vi "File - size rollover.vi"(8 "error in (no error)":errorcluster) -> (0 "error out":errorcluster)   [LabVIEW 2026, in "Tests.lvlib"]
doc: "Integration test (Caraya). Verifies a statement logged through the Logger reaches a single registered appender. Launches a manager with the default file disabled and a queue-mode relay capture probe (Open Test Mgr), logs one INFO statement, dequeues from the capture queue with a timeout, and asserts it was delivered and its message matches. Tears down with Close Test Mgr regardless of assertion outcome (SRS-LMBR-019). Uses the manager fixture; no temp root needed.\n\nImplements LMBR-T-039 -> SRS-033. Assert-level IDs: Test-ID-Assert-Checklist.md."
uses:
  Tests.lvlib
  src/TypeDefs/Severity.ctl
  src/TypeDefs/FileAppenderConfig.ctl
  src/TypeDefs/AppenderConfig.ctl
  src/TypeDefs/Filter.ctl
  src/TypeDefs/FilterMode.ctl
  src/TypeDefs/DropPolicy.ctl
  src/TypeDefs/FileConfig.ctl
  <vilib>/addons/_JKI Toolkits/Caraya/classes/Assert/Assert Less_Variant.vi
  <vilib>/addons/_JKI Toolkits/Caraya/classes/Assert/Assert Equal Value_Variant.vi
  <vilib>/addons/_JKI Toolkits/Caraya/classes/Assert/Assert True.vi
  <vilib>/addons/_JKI Toolkits/Caraya/classes/Test/Test.lvclass
  src/Lumberjack.lvlib
  src/Public/Logger.lvclass/Logger.lvclass
  <vilib>/addons/_JKI Toolkits/Caraya/classes/Assert/Assert.lvclass
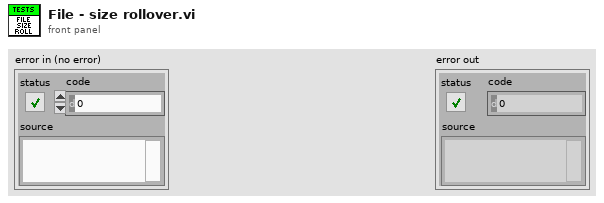
[diagram p1: front panel]
types:
  T1 = typedef "Lumberjack.lvlib/Severity.ctl" = enum16{"OFF", "FATAL", "ERROR", "WARN", "INFO", "DEBUG", "TRACE", "ALL"}
  T2 = typedef "Lumberjack.lvlib/FileAppenderConfig.ctl" = cluster{"common":T3, "file":T7}
  T3 = typedef "Lumberjack.lvlib/AppenderConfig.ctl" = cluster{"id":string, "threshold":T1, "filter":T4, "queueBound":i32, "dropPolicy":T6, "useUTC":bool}
  T4 = typedef "Lumberjack.lvlib/Filter.ctl" = cluster{"mode":T5, "levelMin":T1, "levelMax":T1, "tagPrefix":string}
  T5 = typedef "Lumberjack.lvlib/FilterMode.ctl" = enum16{"Mirror", "Routed"}
  T6 = typedef "Lumberjack.lvlib/DropPolicy.ctl" = enum16{"DropOldest", "DropNewest", "LevelAware"}
  T7 = typedef "Lumberjack.lvlib/FileConfig.ctl" = cluster{"rootFolder":path, "maxFileSize":i64, "maxFileCount":i32, "baseName":string, "extension":string, "delimiter":string, "calendarFolderTree":bool}
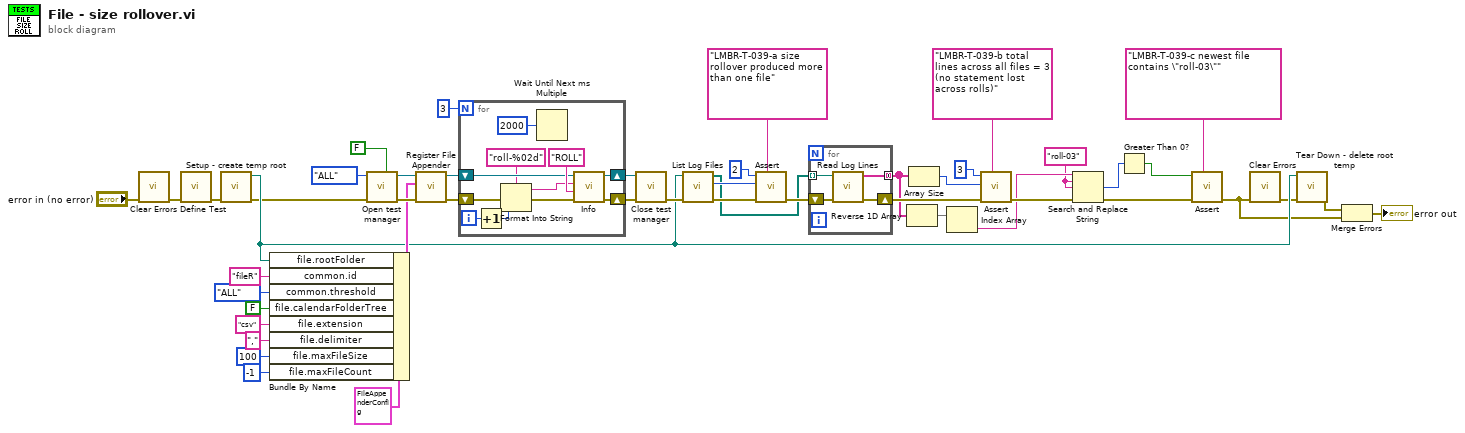
[diagram p0: block diagram]
diagram:
  w10 = "roll-03" ("search string")
  n1 = call <vilib>:"Clear Errors.vi"("error in (no error)"="error in (no error)") -> ("error out"=w5:errorcluster)  [unwired: 5 in, 1 out]
  n2 = call <vilib>:"Define Test.vi"("error in (no error)"=w5) -> ("error out"=w7:errorcluster)  [unwired: 9 in, 1 out]
  n3 = call "Setup - create temp root.vi"("error in (no error)"=w7) -> ("error out"=w24:errorcluster, "tempRoot"=w25:path)  [unwired: 9 in]
  n4 = Bundle By Name(cluster=T2 {"common"={"id"="", "threshold"=enum."INFO", "filter"={"mode"=enum."Mirror", "levelMin"=enum."INFO", "levelMax"=enum."INFO", "tagPrefix"=""}, "queueBound"=0, "dropPolicy"=enum."DropOldest", "useUTC"=FALSE}, "file"={"rootFolder"=path "", "maxFileSize"=0, "maxFileCount"=0, "baseName"="", "extension"="", "delimiter"="", "calendarFolderTree"=FALSE}} ("FileAppenderConfig"), "file.rootFolder"=w25, "common.id"="fileR", "common.threshold"=Severity."ALL", "file.calendarFolderTree"=FALSE, "file.extension"="csv", "file.delimiter"=",", "file.maxFileSize"=i64 100, "file.maxFileCount"=-1) -> (w42:T2)
  n5 = call "Open test manager.vi"("enableDefaultFile"=FALSE, "error in (no error)"=w24, "globalThreshold"=Severity."ALL") -> ("error out"=w45:errorcluster, "Logger out"=w41:refnum<class "Logger.lvclass">)  [unwired: 7 in]
  n6 = call "Register File Appender.vi"("error in (no error)"=w45, "FileAppenderConfig"=w42, "Logger in"=w41) -> ("error out"=w20:errorcluster, "Logger out"=w23:refnum<class "Logger.lvclass">)  [unwired: 6 in, 1 out]
  n7 = for {
    N: 3 -> [_]
    shift-right: [w56] -> w22
    shift-left: w23 -> [w57]
    shift-right: [w55] -> w21
    shift-left: w20 -> [w54]
    i -> [w51]
    n8 = Increment(x=w51) -> (x+1=w50:i32)
    n9 = Format Into String(format string="roll-%02d" ("message"), error in=w54, w50) -> (resulting string=w49:string, error out=w53:errorcluster)  [unwired: 1 in]
    n10 = Wait Until Next ms Multiple(millisecond multiple=u32 2000) -> ()  [unwired: 1 out]
    n11 = call "Info.vi"("error in (no error)"=w53, "sourceTag"="ROLL", "message"=w49, "Logger in"=w57) -> ("error out"=w55:errorcluster, "Logger out"=w56:refnum<class "Logger.lvclass">)  [unwired: 6 in]
  }
  n12 = call "Close test manager.vi"("error in (no error)"=w21, "Logger in"=w22) -> ("error out"=w38:errorcluster)  [unwired: 7 in]
  n13 = call "List Log Files.vi"("error in (no error)"=w38, "rootFolder"=w25) -> ("error out"=w36:errorcluster, "count"=w37:i32, "filePaths"=w18:path[])  [unwired: 7 in]
  n14 = call-poly <vilib>:"Assert.vi"("Label"="LMBR-T-039-a size rollover produced more than one file", "error in (no error)"=w36, "Actual"=w37, "Expected"=2) -> ("error out"=w29:errorcluster)  [unwired: 6 in, 1 out]
  n15 = for {
    tunnel: [w60] -> w15 mode=concatenating
    shift-right: [w61] -> w17
    shift-left: w29 -> [w62]
    tunnel: w18 -> [w59] mode=indexing
    n16 = call "Read Log Lines.vi"("error in (no error)"=w62, "filePath"=w59) -> ("error out"=w61:errorcluster, "lines"=w60:string[])  [unwired: 8 in]
  }
  n17 = Reverse 1D Array(array=w15) -> (reversed array=w14:string[])
  n18 = Array Size(array=w15) -> (size(s)=w16:i32)
  n19 = Index Array(array=w14) -> (element=w11:string)  [unwired: 1 in]
  n20 = call-poly <vilib>:"Assert.vi"("Label"="LMBR-T-039-b total lines across all files = 3 (no statement lost across rolls)", "error in (no error)"=w17, "Actual"=w16, "Expected"=3) -> ("error out"=w13:errorcluster)  [unwired: 6 in, 1 out]
  n21 = Search and Replace String(input string=w11, search string=w10, replace string=w10, error in=w13) -> (number of replacements=w9:i32, error out=w12:errorcluster)  [unwired: 4 in, 2 out]
  n22 = Greater Than 0?(x=w9) -> (x > 0?=w8:bool)
  n23 = call-poly <vilib>:"Assert.vi"("Label"="LMBR-T-039-c newest file contains \"roll-03\"", "error in (no error)"=w12, "True?"=w8) -> ("error out"=w3:errorcluster)  [unwired: 7 in, 1 out]
  n24 = call <vilib>:"Clear Errors.vi"("error in (no error)"=w3) -> ("error out"=w4:errorcluster)  [unwired: 5 in, 1 out]
  n25 = call "Tear Down - delete root temp.vi"("error in (no error)"=w4, "tempRoot"=w25) -> ("error out"=w2:errorcluster)  [unwired: 9 in]
  n26 = Merge Errors(w2, w3) -> (→"error out":errorcluster)
